vi "Renishaw-XL80_GetAutoCompensationMode.vi"(8 "error in (no error)":errorcluster, 11 "Renishaw-XL80 in":refnum<class "Renishaw-XL80.lvclass">) -> (0 "error out":errorcluster, 2 "AutoCompensationMode":i32(ring) items=["AUTO_COMPENSATION_OFF"=0, "AUTO_COMPENSATION_AIR"=1, "AUTO_COMPENSATION_FULL"=3], 3 "Renishaw-XL80 out":refnum<class "Renishaw-XL80.lvclass">)   [LabVIEW 2024, in "Renishaw-XL80.lvclass"]
doc: "Reading this property retrieves the current compensation mode.\n\nDefinition\nHRESULT\nget_AutoCompensationMode(\n [out, retval] AUTO_COMPENSATION_MODES* pVal\n);\nParameters\npVal\nA variable that will be set to one of the values in the enumerated type AUTO_COMPENSATION_MODES.\n\nComments\nReading this property will always retrieve the current compensation mode.\n\nThe property will normally return an HRESULT of S_OK. However, it will return E_POINTER if the client supplies a null pointer for pVal."
uses:
  Renishaw-XL80.lvclass
  Renishaw-XL80.lvclass/Renishaw-XL80.ctl
  D:/A.C.M/Example CSharp_64/bin/Debug/Interop.DX10SDKADAPTORLib.dll
  Example CSharp_64/bin/Debug/Interop.DX10SDKADAPTORLib.dll
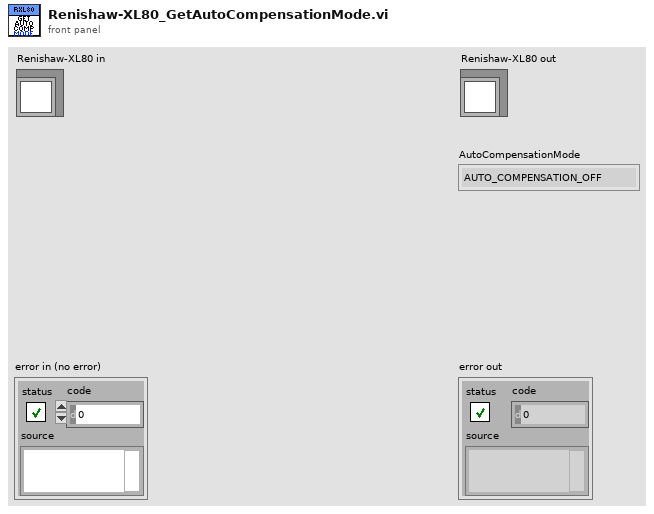
[diagram p1: front panel]
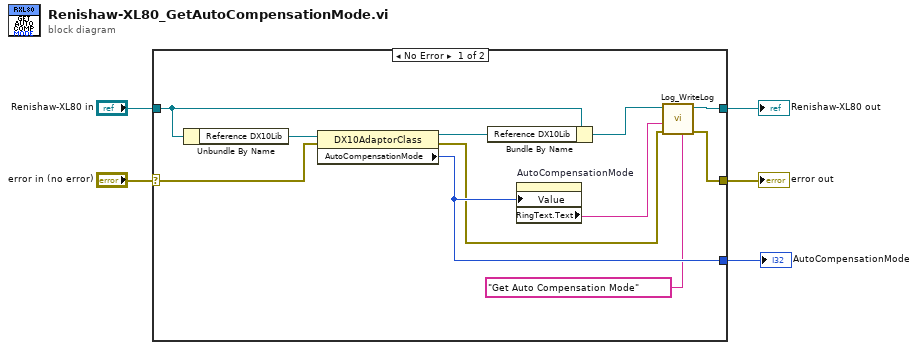
[diagram p0: block diagram]
diagram:
  n1 = case shown="No Error" "error in (no error)" {
    selector: "error in (no error)" -> [w13 w18]
    tunnel: [w10 w18] -> w4
    tunnel: [w11 w17] -> w2
    tunnel: "Renishaw-XL80 in" -> [w14 w17]
    tunnel: [w9 _] -> w1
    frame No Error {
      n2 = Unbundle By Name(w14) -> ("Reference DX10Lib"=w16:refnum<k24>)
      n3 = property class="DX10AdaptorClass"(reference=w16, error in=w13) -> (reference out=w15:refnum<k24>, error out=w6:errorcluster, "AutoCompensationMode"=w9:i32)
      n4 = Bundle By Name(cluster=w14, "Reference DX10Lib"=w15) -> (w12:refnum<class "Renishaw-XL80.lvclass">)
      n5 = property on="AutoCompensationMode" class="Ring (strict)"("Value"=w9) -> ("RingText.Text"=w8:string)  [unwired: 2 in, 2 out]
      n6 = call-dynamic "Log_WriteLog.vi"("Additional text"="Get Auto Compensation Mode", "error in (no error)"=w6, "Response"=w8, "Log in"=w12) -> ("error out"=w10:errorcluster, "Log out"=w11:refnum<class "Renishaw-XL80.lvclass">)  [unwired: 6 in]
    }
    frame Error {
    }
  }
  "error out" <- w4
  "Renishaw-XL80 out" <- w2
  "AutoCompensationMode" <- w1
